vi "Delete Layer.vi"(8 "error in (no error)":errorcluster, 9 "Layer Index":i32, 11 "Image in":refnum<class "Image.lvclass">) -> (0 "error out":errorcluster, 3 "Image out":refnum<class "Image.lvclass">)   [LabVIEW 2017, in "LV Image Editor Framework.lvlib" / "Image.lvclass"]
uses:
  Image.lvclass
  Image.lvclass/Image.ctl
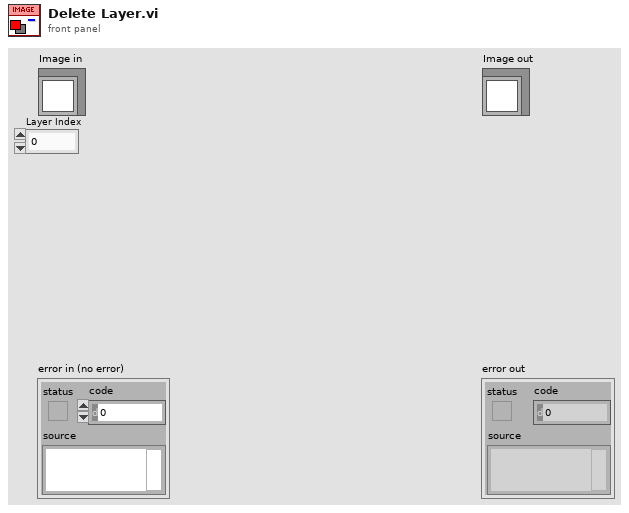
[diagram p1: front panel]
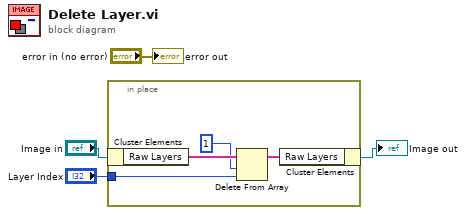
[diagram p0: block diagram]
diagram:
  n1 = in-place {
    in-place-border: "Layer Index" -> [w5]
    n2 = in-place-cluster #1("Image in") -> ("Raw Layers"=w8:string[])
    n3 = Delete From Array(array=w8, length=1, index=w5) -> (array with subset deleted=w7:string[])  [unwired: 1 out]
    n4 = in-place-cluster #1("Raw Layers"=w7) -> (→"Image out":refnum<class "Image.lvclass">)
  }
  "error out" <- "error in (no error)"
